vi "Initialize.vi"(7 "Serial Configuration":T1={"Baud Rate"=9600, "Parity"=0, "Data Bits"=8, "Stop Bits"=10, "Flow Control"=0} {"Flow Control" items=["None", "XON/XOFF", "RTS/CTS", "XON/XOFF & RTS/CTS", "DTR/DSR", "XON/XOFF & DTR/DSR"]; "Stop Bits" items=["1.0"=10, "1.5"=15, "2.0"=20]; "Data Bits" items=["7"=7, "8"=8]; "Parity" items=["None", "Odd", "Even", "Mark", "Space"]; "Baud Rate" items=["300"=300, "600"=600, "1200"=1200, "2400"=2400, "4800"=4800, "9600"=9600, "19200"=19200]}, 8 "error in (no error)":errorcluster, 9 "Reset (True)":bool=TRUE, 10 "ID Query (True)":bool=TRUE, 11 "VISA resource name":refnum<visa-resource-name>) -> (0 "error out":errorcluster, 3 "VISA resource name out":refnum<visa-resource-name>)   [LabVIEW 2019, in "Keithley 2600 Series.lvlib"]
doc: "Establishes communication with the instrument and optionally performs an instrument identification query and/or an instrument reset. It also places the instrument in a default state needed for other instrument driver operations. Therefore, call this VI before calling other instrument driver VIs for this instrument. Generally, you need to call the <b>Initialize</b> VI only once at the beginning of an application."
uses:
  Keithley 2600 Series.lvlib
panel:
  # "(c) 2020 - 2022 National Instruments.  ALL RIGHTS RESERVED."
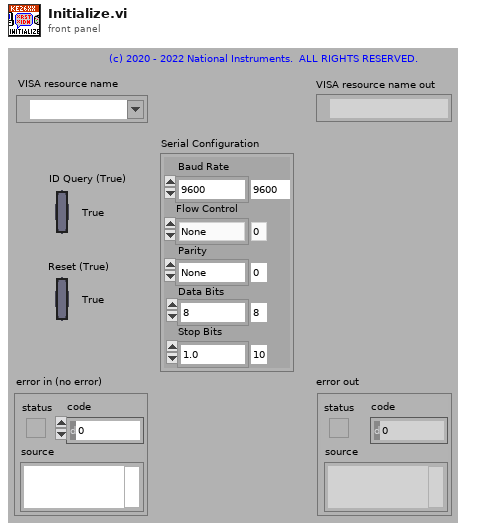
[diagram p1: front panel]
types:
  T1 = cluster{"Baud Rate":u32, "Parity":u16, "Data Bits":u16, "Stop Bits":u16, "Flow Control":u16}
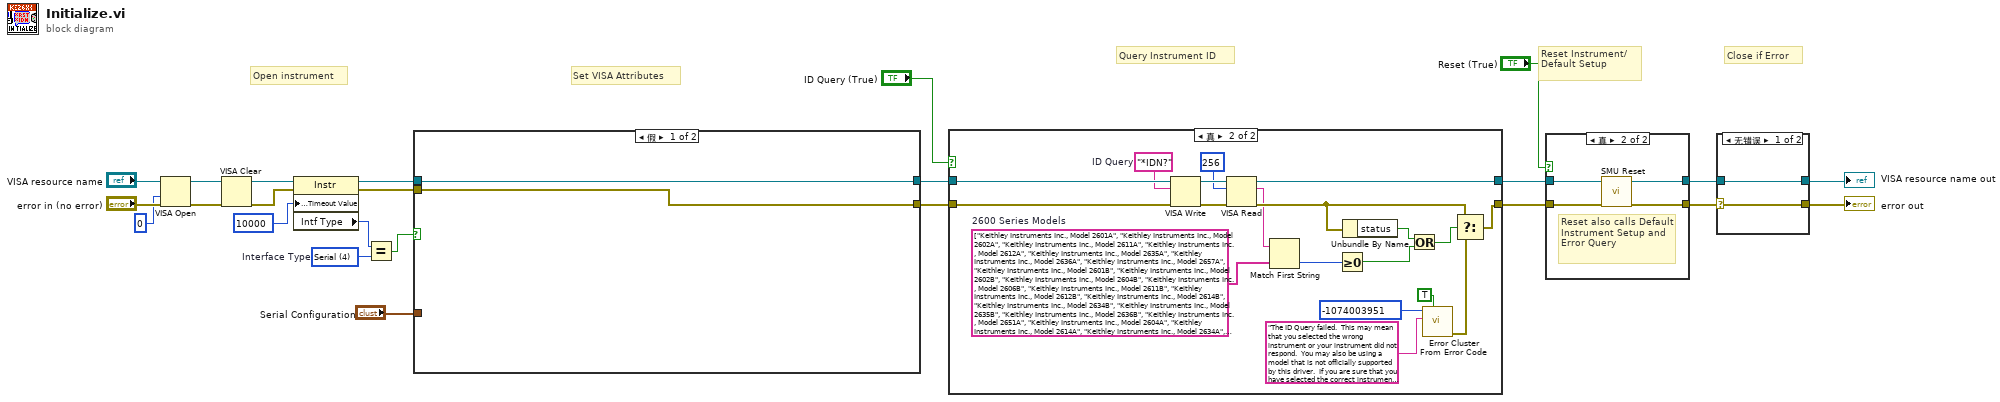
[diagram p0: block diagram]
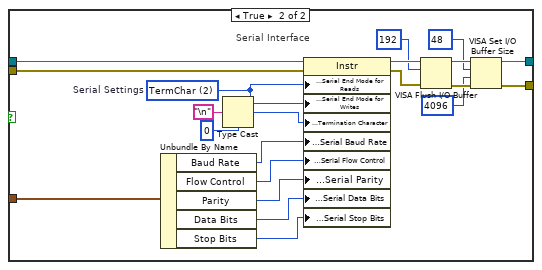
[diagram p2: hidden frame]
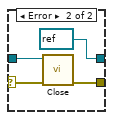
[diagram p3: hidden frame]
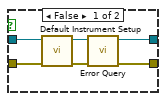
[diagram p4: hidden frame]
diagram:
  w8 = u16 4 items=["GPIB"=1, "VXI"=2, "GPIB-VXI"=3, "Serial"=4, "PXI"=5, "TCPIP"=6, "USB"=7]  # Interface Type
  # "Set VISA Attributes"
  # "Close if Error"
  # "Query Instrument ID"
  # "Reset Instrument/\nDefault Setup"
  # "Open instrument"
  n1 = VISA Open(access mode=u32 0, error in (no error)="error in (no error)", VISA resource name="VISA resource name") -> (VISA resource name=w16:refnum<visa-resource-name>, error out=w15:errorcluster)  [unwired: 2 in]
  n2 = VISA Clear(VISA resource name=w16, error in (no error)=w15) -> (VISA resource name out=w14:refnum<visa-resource-name>, error out=w13:errorcluster)
  n3 = property class="Instr"(reference=w14, error in=w13, "General Settings:Timeout Value"=u32 10000) -> (reference out=w6:refnum<visa-resource-name>, error out=w5:errorcluster, "Intf Type"=w7:u16)
  n4 = Equal?(x=w7, y=w8) -> (x = y?=w2:bool)
  n5 = case shown="假" w2 {
    tunnel: [w25 w44] -> w4
    tunnel: [w26 w41] -> w3
    tunnel: w6 -> [w25 w46]
    tunnel: w5 -> [w26 w47]
    tunnel: "Serial Configuration" -> [_ w27]
    frame False {
    }
    frame True {
      w34 = u16 2 items=["None", "LastBit", "TermChar"]  # Serial Settings
      # "Serial Interface"
      n6 = Unbundle By Name(w27) -> ("Baud Rate"=w32:u32, "Flow Control"=w29:u16, "Parity"=w30:u16, "Data Bits"=w31:u16, "Stop Bits"=w28:u16)
      n7 = Type Cast(type=u8 0, x="\n" ("Line Feed Constant")) -> (*(type *) &x=w33:u8)
      n8 = property class="Instr"(reference=w46, error in=w47, "Serial Settings:Serial End Mode for Reads"=w34, "Serial Settings:Serial End Mode for Writes"=w34, "Message Based Settings:Termination Character"=w33, "Serial Settings:Serial Baud Rate"=w32, "Serial Settings:Serial Flow Control"=w29, "Serial Settings:Serial Parity"=w30, "Serial Settings:Serial Data Bits"=w31, "Serial Settings:Serial Stop Bits"=w28) -> (reference out=w40:refnum<visa-resource-name>, error out=w43:errorcluster)
      n9 = VISA Flush I/O Buffer(VISA resource name=w40, mask (16)=u16 192, error in (no error)=w43) -> (VISA resource name out=w45:refnum<visa-resource-name>, error out=w42:errorcluster)
      n10 = VISA Set I/O Buffer Size(VISA resource name=w45, mask (16)=u16 48, size (4096)=u32 4096 ("size (0)"), error in (no error)=w42) -> (VISA resource name out=w44:refnum<visa-resource-name>, error out=w41:errorcluster)
    }
  }
  n11 = case shown="真" "ID Query (True)" {
    tunnel: [w48 w68] -> w23
    tunnel: [w49 w65] -> w24
    tunnel: w4 -> [w49 w66]
    tunnel: w3 -> [w48 w67]
    frame False {
    }
    frame True {
      w51 = string[] ["Keithley Instruments Inc., Model 2601A", "Keithley Instruments Inc., Model 2602A", "Keithley Instruments Inc., Model 2611A", "Keithley Instruments Inc., Model 2612A", "Keithley Instruments Inc., Model 2635A", "Keithley Instruments Inc., Model 2636A", "Keithley Instruments Inc., Model 2657A", "Keithley Instruments Inc., Model 2601B", "Keithley Instruments Inc., Model 2602B", "Keithley Instruments Inc., Model 2604B", "Keithley Instruments Inc., Model 2606B", "Keithley Instruments Inc., Model 2611B", "Keithley Instruments Inc., Model 2612B", "Keithley Instruments Inc., Model 2614B", "Keithley Instruments Inc., Model 2634B", "Keithley Instruments Inc., Model 2635B", "Keithley Instruments Inc., Model 2636B", "Keithley Instruments Inc., Model 2651A", "Keithley Instruments Inc., Model 2604A", "Keithley Instruments Inc., Model 2614A", "Keithley Instruments Inc., Model 2634A", "Keithley Instruments, Model 2601B-PULSE"]  # 2600 Series Models
      w61 = "*IDN?"  # ID Query
      n12 = VISA Write(VISA resource name=w66, write buffer=w61, error in (no error)=w67) -> (VISA resource name out=w64:refnum<visa-resource-name>, error out=w63:errorcluster)  [unwired: 1 out]
      n13 = VISA Read(VISA resource name=w64, byte count=u32 256, error in (no error)=w63) -> (VISA resource name out=w65:refnum<visa-resource-name>, read buffer=w50:string, error out=w56:errorcluster)  [unwired: 1 out]
      n14 = Match First String(2:w51, 3:w50) -> (0:w52:i32)  [unwired: 1 out]
      n15 = Greater Or Equal To 0?(x=w52) -> (x >= 0?=w54:bool)
      n16 = Unbundle By Name(w56) -> ("status"=w55:bool)
      n17 = Or(x=w55, y=w54) -> (x .or. y?=w53:bool)
      n18 = call <vilib>:"Error Cluster From Error Code.vi"("show call chain? (False)"=TRUE, "error message (\"\")"="The ID Query failed.  This may mean that you selected the wrong instrument or your instrument did not respond.  You may also be using a model that is not officially supported by this driver.  If you are sure that you have selected the correct instrument and it is responding, try disabling the ID Query." ("Source (VI Name)"), "error code (0)"=-1074003951 ("Code")) -> ("error out"=w60:errorcluster)  [unwired: 6 in]
      n19 = Select(t=w56, s=w53, f=w60) -> (s? t:f=w68:errorcluster)
    }
  }
  n20 = case shown="真" "Reset (True)" {
    tunnel: w23 -> [w73 w76]
    tunnel: [w70 w75] -> w9
    tunnel: w24 -> [w74 w78]
    tunnel: [w71 w77] -> w10
    frame False {
      n21 = call "Default Instrument Setup.vi"("error in (no error)"=w73, "VISA resource name"=w74) -> ("error out"=w69:errorcluster, "VISA resource name out"=w72:refnum<visa-resource-name>)  [unwired: 8 in]
      n22 = call "Error Query.vi"("error in (no error)"=w69, "VISA resource name"=w72) -> ("error out"=w70:errorcluster, "VISA resource name out"=w71:refnum<visa-resource-name>)  [unwired: 6 in, 2 out]
    }
    frame True {
      # "Reset also calls Default Instrument Setup and Error Query"
      n23 = call "SMU Reset.vi"("error in (no error)"=w76, "VISA resource name"=w78) -> ("error out"=w75:errorcluster, "VISA resource name out"=w77:refnum<visa-resource-name>)  [unwired: 8 in]
    }
  }
  n24 = case shown="无错误" w9 {
    selector: w9 -> [w79 w82]
    tunnel: w10 -> [w80 w83]
    tunnel: [w80 refnum<visa-resource-name> refnum ("VISA resource name out")] -> w12
    tunnel: [w79 w84] -> w11
    frame No Error {
    }
    frame Error {
      n25 = call "Close.vi"("error in (no error)"=w82, "VISA resource name"=w83) -> ("error out"=w84:errorcluster)  [unwired: 9 in]
    }
  }
  "VISA resource name out" <- w12
  "error out" <- w11
